vi "OpenVI.vi"(0 "CloneRef":refnum<vi>, 1 "OpenFP":bool, 2 "Vi_relative_Path":string) -> (3 "ResponseXML":string, 4 "ControlIndicator":T1(array[cluster]), 5 "vi reference":refnum<vi>, 6 "OpenedOK?":bool)   [LabVIEW 2010]
panel:
  out "error out 2":errorcluster
  out "error out 5":errorcluster
  out "ArrayOfStructsXML":string
  out "error out":errorcluster
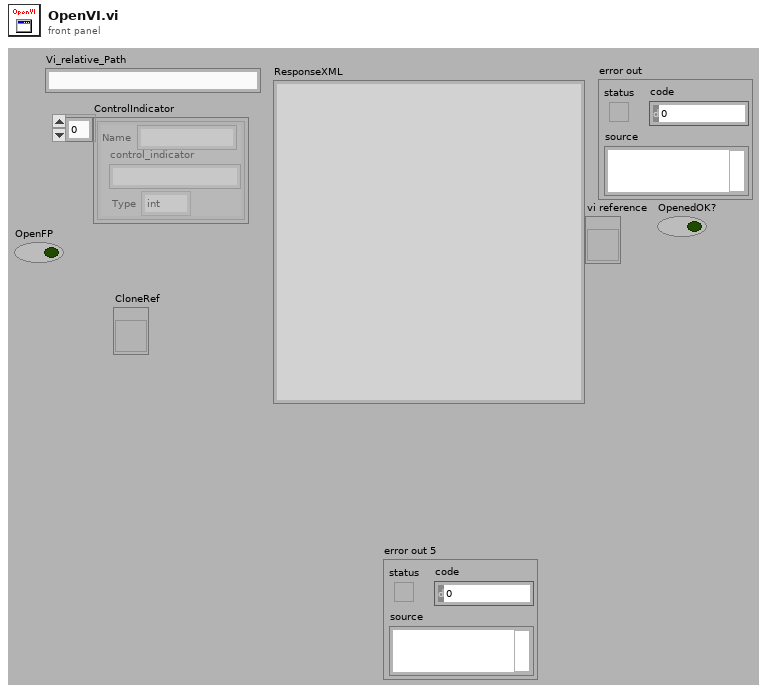
[diagram p1: front panel]
types:
  T1 = cluster{"Name":string, "control_indicator":string, "Type":enum16{"int", "boolean", "string", "double", "dateTime", "base64", "struct", "array"}}[]
  T2 = cluster{"Name":string, string, "Type":enum16{"int", "boolean", "string", "double", "dateTime", "base64", "struct", "array"}}[]
  T3 = enum16{"Update", "registry", "Init", "clean", "Close"}
  T4 = enum32{"Bad", "Idle", "Run top level", "Running"}
  T5 = enum32{"Invalid", "Standard", "Closed", "Hidden", "Minimized", "Maximized"}
  T6 = enum16{"int", "boolean", "string", "double", "dateTime", "base64", "struct", "array"}
  T7 = cluster{"Name":string, string, "Type":enum16{"int", "boolean", "string", "double", "dateTime", "base64", "struct", "array"}}
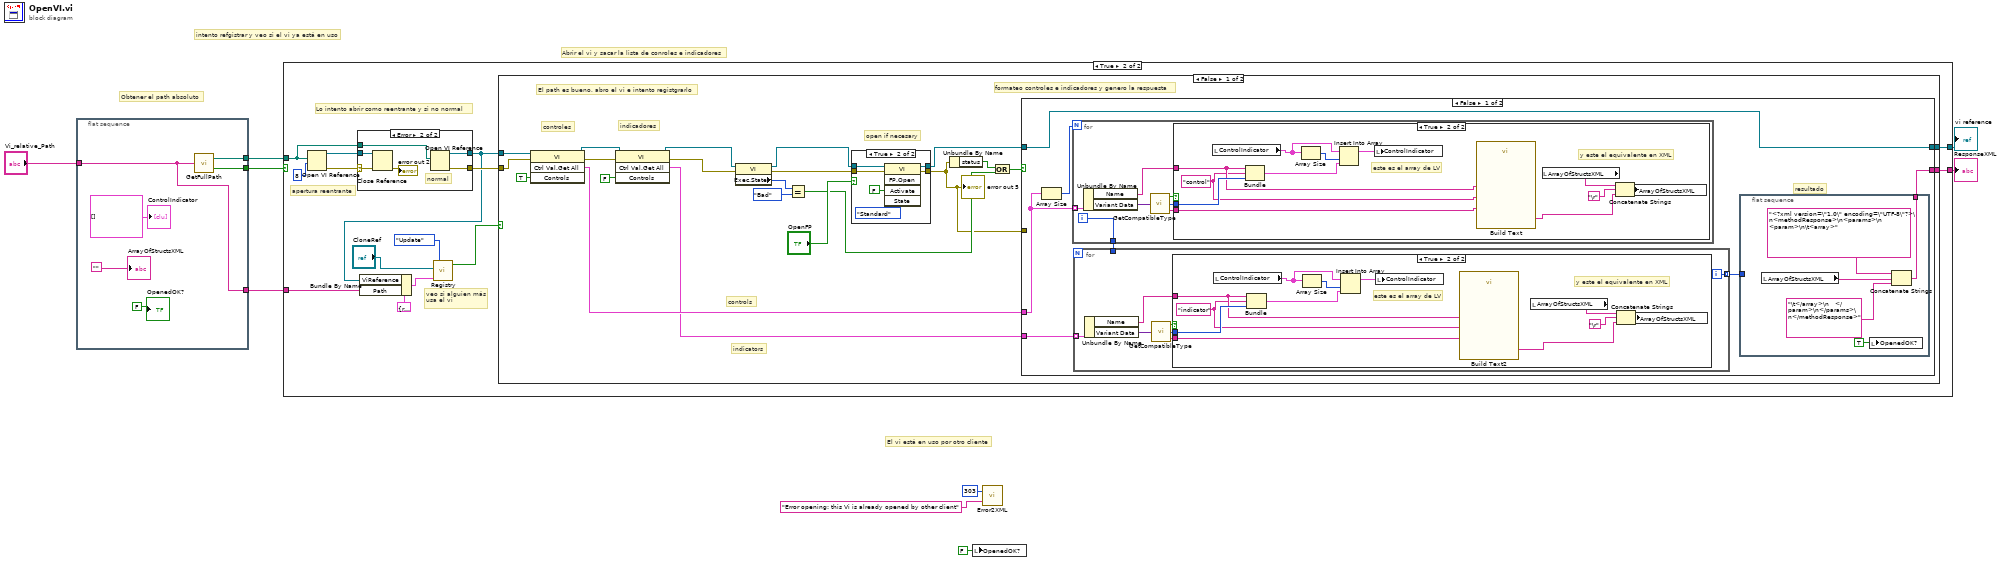
[diagram p0: block diagram]
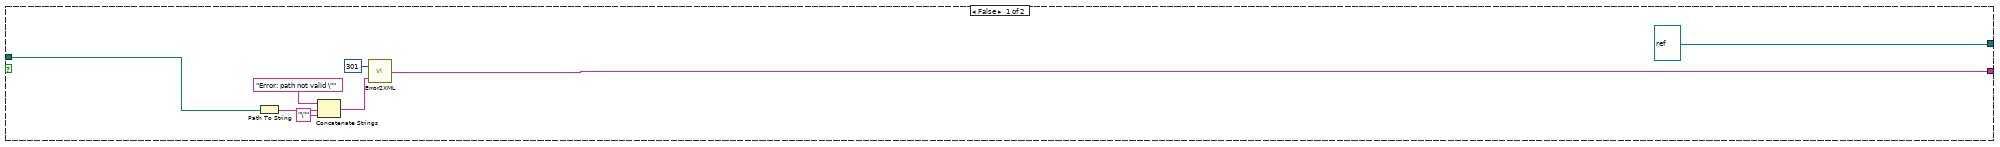
[diagram p2: hidden frame]
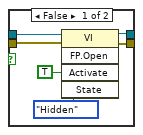
[diagram p3: hidden frame]
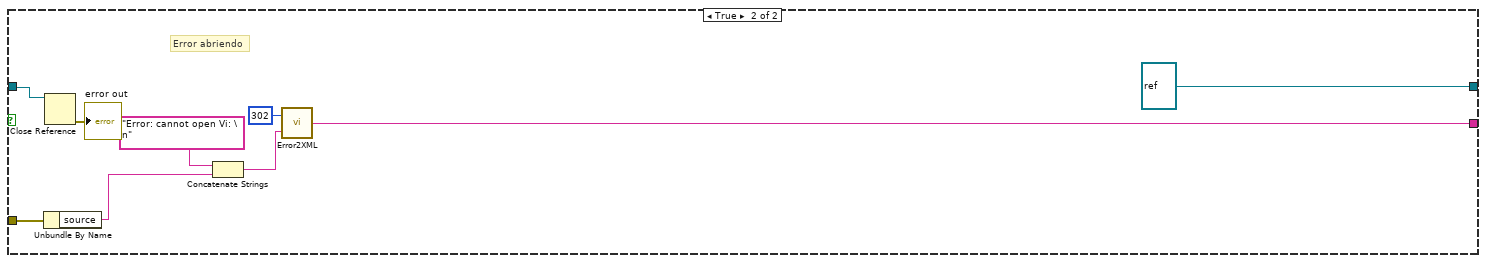
[diagram p6: hidden frame]
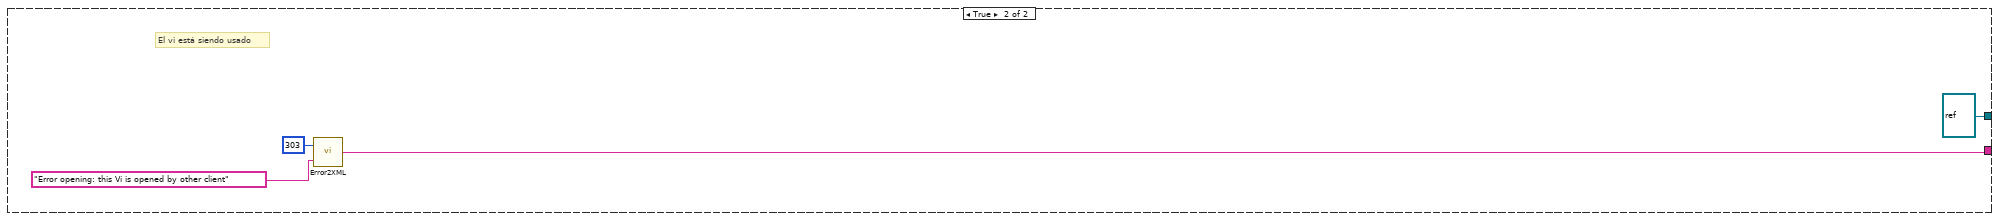
[diagram p7: hidden frame]
diagram:
  # "Abrir el vi y sacar la lista de conroles e indicadores"
  # "Obtener el path absoluto"
  # "El vi está en uso por otro cliente"
  # "intento refgistrar y veo si el vi ya está en uso"
  n1 = flat-sequence {
    tunnel: [w15] -> w3
    tunnel: [w14] -> w2
    tunnel: "Vi_relative_Path" -> [w10]
    tunnel: [w10] -> w1
    frame #0 {
      n2 = call "GetFullPath.vi"("string Path in"=w10) -> ("Path is Ok?"=w15:bool, "absolute path"=w14:path)
      "ControlIndicator" <- T2 [] ("ControlIndicator")
      "ArrayOfStructsXML" <- ""
      "OpenedOK?" <- FALSE
    }
  }
  n3 = case shown="True" w3 {
    tunnel: w2 -> [w19 w29]
    tunnel: [w17 w36] -> w9
    tunnel: [refnum<vi> refnum ("vi reference") w37] -> w8
    tunnel: w1 -> [_ w26]
    frame False {
      n4 = Path To String(path=w19) -> (string=w20:string)
      n5 = Concatenate Strings("Error: path not valid \"" ("FailDescriptor"), w20, "\"" ("string")) -> (w21:string)
      n6 = call "Error2XML.vi"("FailDescriptor"=w21, "FailID"=301) -> ("ErrorXML"=w17:string)
    }
    frame True {
      # "apertura reentrante"
      # "Lo intento abrir como reentrante y si no normal"
      # "veo si alguien más\nusa el vi"
      n7 = Open VI Reference(vi path=w29, options=8) -> (vi reference=w31:refnum<vi>, error out=w32:errorcluster)  [unwired: 2 in, 2 out]
      n8 = case shown="Error" w32 {
        selector: w32 -> [w135 w141]
        tunnel: [w136 w140] -> w25
        tunnel: w31 -> [w136 w142]
        tunnel: [w135 w139] -> w30
        tunnel: w29 -> [_ w138]
        frame No Error {
        }
        frame Error {
          # "normal"
          n9 = Close Reference(reference=w142, error in (no error)=w141) -> (error out=→"error out 2":errorcluster)
          n10 = Open VI Reference(vi path=w138) -> (vi reference=w140:refnum<vi>, error out=w139:errorcluster)  [unwired: 2 in, 3 out]
        }
      }
      n11 = Bundle By Name(cluster=cluster{"ViReference":refnum<vi>, "Path":string} {"ViReference"=refnum, "Path"=""} ("OpenedVI"), "ViReference"=w25, "Path"=w26) -> (w27:cluster{"ViReference":refnum<vi>, "Path":string})
      n12 = call "Registry.vi"("OpenedVI"=w27, "ParserReferecne"="CloneRef", "Command"=T3."Update") -> ("VI_in_use?"=w24:bool)  [unwired: 1 in, 2 out]
      n13 = case shown="False" w24 {
        tunnel: [w59 refnum<vi> refnum ("vi reference")] -> w37
        tunnel: [w58 w132] -> w36
        tunnel: w25 -> [w39 _]
        tunnel: w30 -> [w38 _]
        frame False {
          # "open if necesary"
          # "indicators"
          # "controls"
          # "formateo controles e indicadores y genero la respuesta"
          # "indicadores"
          # "controles"
          # "El path es bueno, abro el vi e intento registgrarlo"
          n14 = invoke class="VI" method="Ctrl Val.Get All"(reference=w39, error in=w38, "Controls"=TRUE) -> (reference out=w56:refnum<vi>, error out=w55:errorcluster, "Get All Control Values Variant"=w53:cluster{"Name":string, "Variant Data":variant}[])  [unwired: 1 in, 1 out]
          n15 = invoke class="VI" method="Ctrl Val.Get All"(reference=w56, error in=w55, "Controls"=FALSE) -> (reference out=w46:refnum<vi>, error out=w51:errorcluster, "Get All Control Values Variant"=w52:cluster{"Name":string, "Variant Data":variant}[])  [unwired: 1 in, 1 out]
          n16 = property class="VI"(reference=w46, error in=w51) -> (reference out=w45:refnum<vi>, error out=w47:errorcluster, "Exec.State"=w50:T4)
          n17 = Equal?(x=w50, y=T4."Bad") -> (x = y?=w42:bool)
          n18 = case shown="True" "OpenFP" {
            tunnel: w45 -> [w62 w71]
            tunnel: w47 -> [w63 w70]
            tunnel: [w64 w69] -> w40
            tunnel: [w65 w68] -> w44
            frame False {
              n19 = invoke class="VI" method="FP.Open"(reference=w62, error in=w63, "Activate"=TRUE ("Activate?"), "State"=T5."Hidden") -> (reference out=w65:refnum<vi>, error out=w64:errorcluster)  [unwired: 1 in, 3 out]
            }
            frame True {
              n20 = invoke class="VI" method="FP.Open"(reference=w71, error in=w70, "Activate"=FALSE ("Activate?"), "State"=T5."Standard") -> (reference out=w68:refnum<vi>, error out=w69:errorcluster)  [unwired: 1 in, 3 out]
            }
          }
          "error out 5" <- w40
          n21 = Unbundle By Name(w40) -> ("status"=w41:bool)
          n22 = Or(x=w41, y=w42) -> (x .or. y?=w43:bool)
          n23 = case shown="False" w43 {
            tunnel: [w74 refnum<vi> refnum ("vi reference")] -> w59
            tunnel: w44 -> [w74 w124]
            tunnel: [w72 w127] -> w58
            tunnel: w53 -> [w77 _]
            tunnel: w52 -> [w76 _]
            tunnel: w40 -> [_ w123]
            frame False {
              # "resultado"
              n24 = Array Size(array=w77) -> (size(s)=w78:i32)
              n25 = for {
                N: w78 -> [_]
                tunnel: w77 -> [w109] mode=indexing
                tunnel: [w103] -> w75
                i -> [w103]
                n26 = Unbundle By Name(w109) -> ("Name"=w106:string, "Variant Data"=w108:variant)
                n27 = call "GetCompatibleType.vi"("variant"=w108) -> ("Text_type"=w104:string, "Type"=w105:T6, "Type found?"=w107:bool)
                n28 = case shown="True" w107 {
                  tunnel: w106 -> [_ w113]
                  tunnel: w105 -> [_ w121]
                  tunnel: w104 -> [_ w111]
                  frame False {
                    # "no hay tipo compatible, paso"
                  }
                  frame True {
                    w112 = "control"
                    # "y este el equivalente en XML"
                    # "este es el array de LV"
                    n29 = local read "ControlIndicator"() -> (w120:T1)
                    n30 = Bundle("Name"=w113, w112, "Type"=w121) -> (w118:T7)  [unwired: 1 in]
                    n31 = Array Size(array=w120) -> (size(s)=w119:i32)
                    n32 = Insert Into Array(array=w120, index=w119, new element=w118) -> (w117:T1)
                    n33 = local write "ControlIndicator"(w117) -> ()
                    n34 = call "Build Text"("name"=w113, "control_indicator"=w112, "DataType"=w111) -> ("Result"=w110:string)  [unwired: 11 in, 1 out]
                    n35 = local read "ArrayOfStructsXML"() -> (w116:string)
                    n36 = Concatenate Strings(w116, "\r", w110) -> (w114:string)
                    n37 = local write "ArrayOfStructsXML"(w114) -> ()
                  }
                }
              }
              n38 = for {
                tunnel: w76 -> [w90] mode=indexing
                tunnel: w75 -> [_]
                tunnel: [w84] -> w73 mode=indexing
                i -> [w84]
                n39 = Unbundle By Name(w90) -> ("Name"=w87:string, "Variant Data"=w89:variant)
                n40 = call "GetCompatibleType.vi"("variant"=w89) -> ("Text_type"=w85:string, "Type"=w86:T6, "Type found?"=w88:bool)
                n41 = case shown="True" w88 {
                  tunnel: w87 -> [_ w101]
                  tunnel: w86 -> [_ w102]
                  tunnel: w85 -> [_ w99]
                  frame False {
                    # "no hay tipo compatible, paso"
                  }
                  frame True {
                    w100 = "indicator"
                    # "y este el equivalente en XML"
                    # "este es el array de LV"
                    n42 = local read "ControlIndicator"() -> (w98:T1)
                    n43 = Bundle("Name"=w101, w100, "Type"=w102) -> (w96:T7)  [unwired: 1 in]
                    n44 = Array Size(array=w98) -> (size(s)=w97:i32)
                    n45 = Insert Into Array(array=w98, index=w97, new element=w96) -> (w95:T1)
                    n46 = local write "ControlIndicator"(w95) -> ()
                    n47 = call "Build Text2"("name"=w101, "control_indicator"=w100, "DataType"=w99) -> ("Result"=w92:string)  [unwired: 11 in, 1 out]
                    n48 = local read "ArrayOfStructsXML"() -> (w94:string)
                    n49 = Concatenate Strings(w94, "\r", w92) -> (w91:string)
                    n50 = local write "ArrayOfStructsXML"(w91) -> ()
                  }
                }
              }
              n51 = flat-sequence {
                tunnel: w73 -> [_]
                tunnel: [w83] -> w72
                frame #0 {
                  n52 = local read "ArrayOfStructsXML"() -> (w81:string)
                  n53 = local write "OpenedOK?"(TRUE ("OpenedOK?")) -> ()
                  n54 = Concatenate Strings("<?xml version=\"1.0\" encoding=\"UTF-8\"?>\n<methodResponse>\n<params>\n     <param>\n\t<array>" ("string"), w81, "\t</array>\n   </param>\n</params>\n</methodResponse>" ("string")) -> (w83:string)
                }
              }
            }
            frame True {
              # "Error abriendo"
              n55 = Unbundle By Name(w123) -> ("source"=w122:string)
              n56 = Close Reference(reference=w124) -> (error out=→"error out":errorcluster)  [unwired: 1 in]
              n57 = Concatenate Strings("Error: cannot open Vi: \n" ("FailDescriptor"), w122) -> (w128:string)
              n58 = call "Error2XML.vi"("FailDescriptor"=w128, "FailID"=302) -> ("ErrorXML"=w127:string)
            }
          }
        }
        frame True {
          # "El vi está siendo usado"
          n59 = call "Error2XML.vi"("FailDescriptor"="Error opening: this Vi is opened by other client", "FailID"=303) -> ("ErrorXML"=w132:string)
        }
      }
    }
  }
  "ResponseXML" <- w9
  "vi reference" <- w8
  n60 = local write "OpenedOK?"(FALSE ("OpenedOK?")) -> ()
  n61 = call "Error2XML.vi"("FailDescriptor"="Error opening: this Vi is already opened by other client", "FailID"=303) -> ()  [unwired: 1 out]
